vi "Configure Trigger (Edge).vi"(0 "VISA resource name":refnum<visa-resource-name>, 5 "Trigger Source (1: Channel1)":i32(ring)=1 items=["Channel1"=1, "Channel2"=2, "Channel3"=3, "Channel4"=4, "AUX"=13, "Line"=14, "DIG0"=20, "DIG1"=21, "DIG2"=22, "DIG3"=23, "DIG4"=24, "DIG5"=25, "DIG6"=26, "DIG7"=27, "DIG8"=28, "DIG9"=29, "DIG10"=30, "DIG11"=31, "DIG12"=32, "DIG13"=33, "DIG14"=34, "DIG15"=35], 9 "Edge Trigger Slope (0: Negative)":i32(ring) items=["Negative", "Positive", "Either"], 11 "error in (no error)":errorcluster) -> (4 "VISA resource name out":refnum<visa-resource-name>, 15 "error out":errorcluster)   [LabVIEW 2013, in "Agilent 90000 Series.lvlib"]
doc: "Configures the edge trigger parameters."
uses:
  Agilent 90000 Series.lvlib
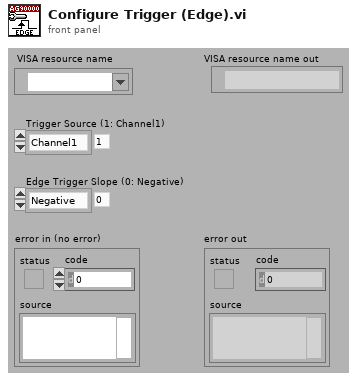
[diagram p1: front panel]
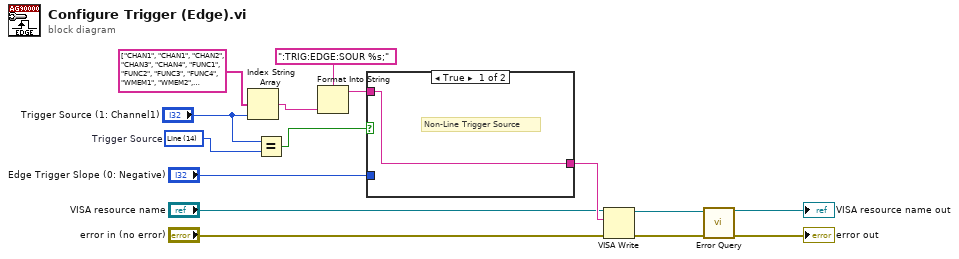
[diagram p0: block diagram]
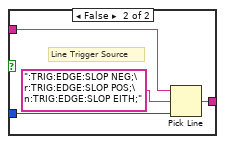
[diagram p2: hidden frame]
diagram:
  w2 = 14 items=["Channel1"=1, "Channel2"=2, "Channel3"=3, "Channel4"=4, "AUX"=13, "Line"=14]  # Trigger Source
  n1 = Index String Array(1:"Trigger Source (1: Channel1)", 2:string[] ["CHAN1", "CHAN1", "CHAN2", "CHAN3", "CHAN4", "FUNC1", "FUNC2", "FUNC3", "FUNC4", "WMEM1", "WMEM2", "WMEM3", "WMEM4", "AUX", "LINE", "CLOC", "MTR", "MSP", "EQU", "NONE", "DIG0", "DIG1", "DIG2", "DIG3", "DIG4", "DIG5", "DIG6", "DIG7", "DIG8", "DIG9", "DIG10", "DIG11", "DIG12", "DIG13", "DIG14", "DIG15", "", "", "", "", "", "POD1", "POD2", "", "", "", "", "", "", "", "", "BUS1", "BUS2", "BUS3", "BUS4", "", "", "", "", "", "", "DIFF1", "DIFF2", "", "", "", "", "", "", "", "", "COMM3", "COMM4"]) -> (0:w4:string)  [unwired: 1 out]
  n2 = Equal?(x="Trigger Source (1: Channel1)", y=w2) -> (x = y?=w1:bool)
  n3 = Format Into String(format string=":TRIG:EDGE:SOUR %s;", w4) -> (resulting string=w7:string)  [unwired: 2 in, 1 out]
  n4 = case shown="True" w1 {
    tunnel: "Edge Trigger Slope (0: Negative)" -> [_ w19]
    tunnel: [w16 w18] -> w14
    tunnel: w7 -> [w16 w17]
    frame True {
      # "Non-Line Trigger Source"
    }
    frame False {
      # "Line Trigger Source"
      n5 = Pick Line(string ("")=w17, multi-line string=":TRIG:EDGE:SLOP NEG;\r:TRIG:EDGE:SLOP POS;\n:TRIG:EDGE:SLOP EITH;", line index=w19) -> (output string=w18:string)
    }
  }
  n6 = VISA Write(VISA resource name="VISA resource name", write buffer=w14, error in (no error)="error in (no error)") -> (VISA resource name out=w11:refnum<visa-resource-name>, error out=w10:errorcluster)  [unwired: 1 out]
  n7 = call "Error Query.vi"("error in (no error)"=w10, "VISA resource name"=w11) -> ("error out"=→"error out":errorcluster, "VISA resource name out"=→"VISA resource name out":refnum<visa-resource-name>)  [unwired: 8 out]
